vi "MKS670_He3_meas_p.vi"(8 "error in":errorcluster, 11 "GPIB Address":string) -> (0 "error out":errorcluster, 1 "status":bool, 2 "msg":string, 3 "value":dbl)   [LabVIEW 2019]
panel:
  out "string 1":string
  out "string 2":string
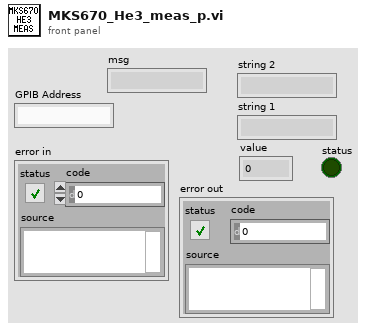
[diagram p1: front panel]
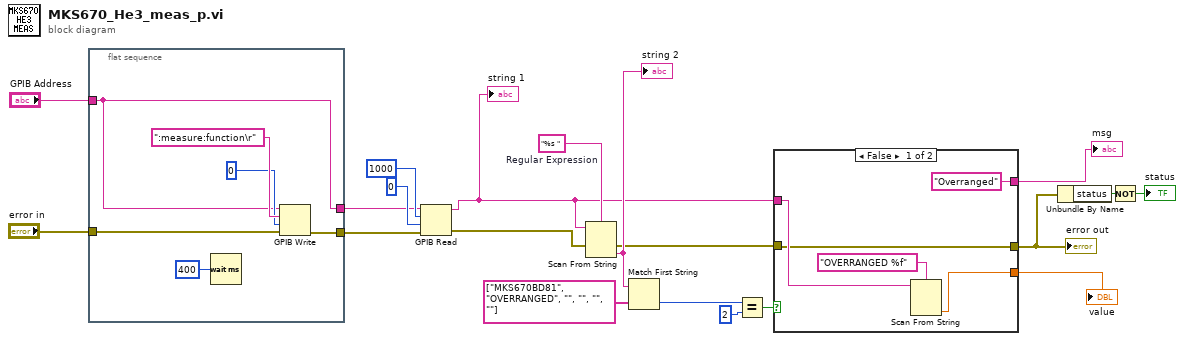
[diagram p0: block diagram]
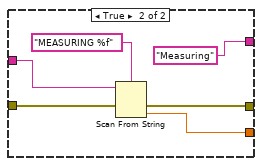
[diagram p2: hidden frame]
diagram:
  w16 = "%s "  # Regular Expression
  n1 = flat-sequence {
    tunnel: [w23] -> w18
    tunnel: [w21] -> w11
    tunnel: "error in" -> [w22]
    tunnel: "GPIB Address" -> [w21]
    frame #0 {
      n2 = Wait (ms)(milliseconds to wait=u32 400) -> ()  [unwired: 1 out]
      n3 = GPIB Write(0:w21, 1:":measure:function\r" ("data"), 2:0, 3:w22) -> (6:w23:errorcluster)  [unwired: 1 in, 1 out]
    }
  }
  n4 = GPIB Read(0:w11, 1:1000 ("byte count"), 2:0, 3:w18) -> (5:w10:string, 7:w9:errorcluster)  [unwired: 1 in, 1 out]
  "string 1" <- w10
  n5 = Scan From String(format string=w16, input string=w10, error in=w9) -> (error out=w7:errorcluster, output 1=w12:string)  [unwired: 2 in, 2 out]
  "string 2" <- w12
  n6 = Match First String(2:string[] ["MKS670BD81", "OVERRANGED", "", "", "", ""], 3:w12) -> (0:w15:i32)  [unwired: 1 out]
  n7 = Equal?(x=w15, y=2) -> (x = y?=w13:bool)
  n8 = case shown="False" w13 {
    tunnel: w10 -> [w31 w37]
    tunnel: [w29 w35] -> w8
    tunnel: [w28 w34] -> w4
    tunnel: w7 -> [w28 w33]
    tunnel: ["Overranged" ("msg") "Measuring" ("msg")] -> w2
    frame False {
      n9 = Scan From String(format string="OVERRANGED %f", input string=w31) -> (output 1=w29:dbl)  [unwired: 3 in, 3 out]
    }
    frame True {
      n10 = Scan From String(format string="MEASURING %f", input string=w37, error in=w33) -> (error out=w34:errorcluster, output 1=w35:dbl)  [unwired: 2 in, 2 out]
    }
  }
  "value" <- w8
  "error out" <- w4
  "msg" <- w2
  n11 = Unbundle By Name(w4) -> ("status"=w3:bool)
  n12 = Not(x=w3) -> (.not. x?=→"status":bool)
